vi "VarMan Compatible Help.vi"(6 "CHM or HLP filename (lvdialog.chm)":string="lvdialog.chm", 7 "error in (no error)":errorcluster, 9 "VarMan HTML Filename":string, 10 "HTML filename":string) -> (0 "error out":errorcluster)   [LabVIEW 2016]
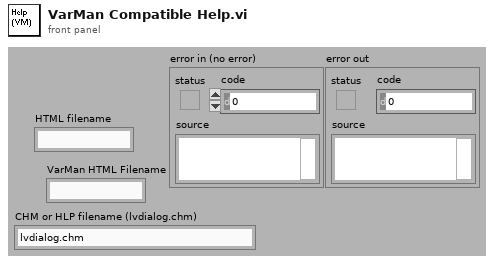
[diagram p1: front panel]
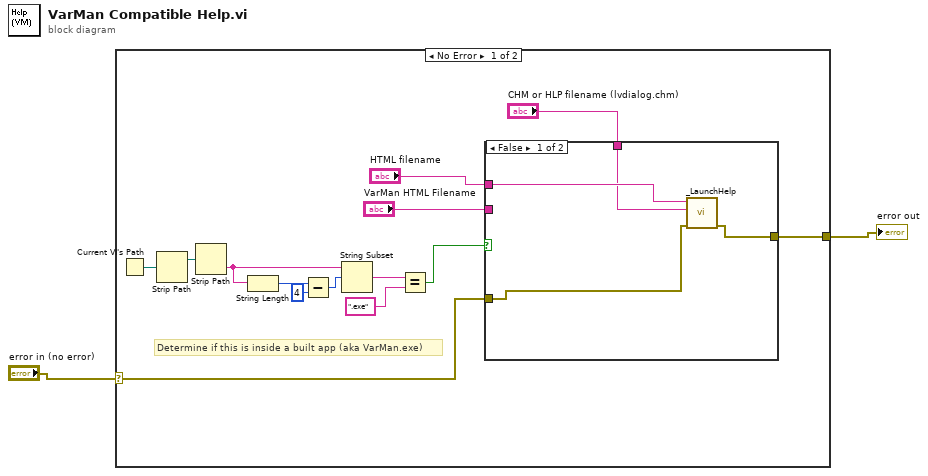
[diagram p0: block diagram]
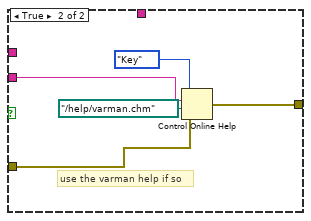
[diagram p2: hidden frame]
diagram:
  n1 = case shown="No Error" "error in (no error)" {
    selector: "error in (no error)" -> [w5 w26]
    tunnel: [w4 w26] -> w1
    frame No Error {
      # "Determine if this is inside a built app (aka VarMan.exe)"
      n2 = Current VI's Path() -> (path=w12:path)
      n3 = Strip Path(path=w12) -> (stripped path=w11:path)  [unwired: 1 out]
      n4 = Strip Path(path=w11) -> (name=w14:string)  [unwired: 1 out]
      n5 = String Length(string=w14) -> (length=w7:i32)
      n6 = Subtract(x=w7, y=4) -> (x-y=w6:i32)
      n7 = String Subset(string=w14, offset (0)=w6) -> (substring=w9:string)  [unwired: 1 in]
      n8 = Equal?(x=w9, y=".exe") -> (x = y?=w13:bool)
      n9 = case shown="False" w13 {
        tunnel: "HTML filename" -> [w20 _]
        tunnel: "VarMan HTML Filename" -> [_ w23]
        tunnel: w5 -> [w19 w22]
        tunnel: [w18 w21] -> w4
        tunnel: "CHM or HLP filename (lvdialog.chm)" -> [w17 _]
        frame False {
          n10 = call <helpdir>:"_LaunchHelp.vi"("error in (no error)"=w19, "CHM or HLP filename (lvdialog.chm)"=w17, "HTML filename"=w20) -> ("error out"=w18:errorcluster)  [unwired: 4 in]
        }
        frame True {
          # "use the varman help if so"
          n11 = Control Online Help(1:w22, 2:path "../help/varman.chm" ("Path to the help file"), 3:w23, 4:enum16{"Contents", "Key", "Close"}."Key" ("Operation")) -> (0:w21:errorcluster)
        }
      }
    }
    frame Error {
    }
  }
  "error out" <- w1
